vi "Plot class probabilities calculated by the VotingClassifier.vi"() -> ()   [LabVIEW 2020]
doc: "Plot the class probabilities of the first sample in a toy dataset predicted by three different classifiers and averaged by the VotingClassifier.\n\nFirst, three examplary classifiers are initialized (LogisticRegression, GaussianNB, and RandomForestClassifier) and used to initialize a soft-voting VotingClassifier with weights [1, 1, 5], which means that the predicted probabilities of the RandomForestClassifier count 5 times as much as the weights of the other classifiers when the averaged probability is calculated.\n\nTo visualize the probability weighting, we fit each classifier on the training set and plot the predicted class probabilities for the first sample in this example dataset."
uses:
  Model/Supervised/Linear_model/LinearClassifiers/LogisticRegression/LogisticRegression.lvclass
  C:/Users/cipop/TDF Dropbox/2_Technologies de France/1 - Services et Etudes/PLAIY/2 - DEV/PLAIYLAB/code/Model/Model.lvclass
  C:/Users/cipop/TDF Dropbox/2_Technologies de France/1 - Services et Etudes/PLAIY/2 - DEV/PLAIYLAB/code/Model/Supervised/Supervised.lvclass
  Model/Supervised/Ensemble/EnsembleClassifier/RandomForestClassifier/RandomForestClassifier.lvclass
  C:/Users/cipop/TDF Dropbox/2_Technologies de France/1 - Services et Etudes/PLAIY/2 - DEV/PLAIYLAB/code/Model/Supervised/Ensemble/Ensemble.lvclass
  Model/Supervised/Naive_bayes/GaussianNB/GaussianNB.lvclass
  C:/Users/cipop/TDF Dropbox/2_Technologies de France/1 - Services et Etudes/PLAIY/2 - DEV/PLAIYLAB/code/Model/Supervised/Naive_bayes/Naive_bayes.lvclass
  Model/Supervised/Linear_model/LinearClassifiers/LogisticRegression/Controls/logistic_regression_params.ctl
  Model/Supervised/Ensemble/EnsembleClassifier/RandomForestClassifier/Controls/random_forest_classifier_params.ctl
  Model/Supervised/Naive_bayes/GaussianNB/Controls/gaussian_nb_params.ctl
  Model/Supervised/Ensemble/EnsembleBlender/VotingClassifier/Controls/voting_classifier_params.ctl
  Model/Supervised/Supervised.lvclass
  Model/Supervised/Ensemble/EnsembleBlender/VotingClassifier/VotingClassifier.lvclass
  Model/Supervised/Linear_model/LinearClassifiers/LogisticRegression/LogisticRegression.vi
  Model/Supervised/Ensemble/EnsembleClassifier/RandomForestClassifier/RandomForestClassifier.vi
  Model/Supervised/Naive_bayes/GaussianNB/GaussianNB.vi
  Model/Supervised/Ensemble/EnsembleBlender/VotingClassifier/VotingClassifier.vi
panel:
  out "Plot":cluster{"X":dbl[], "Y":dbl[]}[](graph) caption="Class probabilities for sample 1 by different classifiers"
  out "error out":errorcluster
  in  "error in":errorcluster
  in  "Local":T1
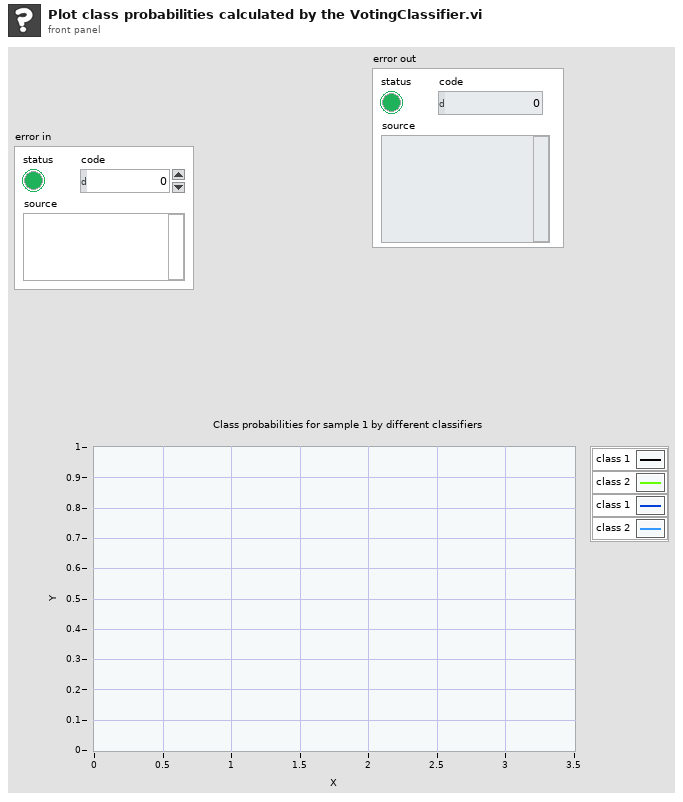
[diagram p1: front panel]
types:
  T1 = cluster{"X":dbl[][], "y":dbl[], "LogisticRegression":refnum<class "LogisticRegression.lvclass">, "RandomForestClassifier":refnum<class "RandomForestClassifier.lvclass">, "GaussianNB":refnum<class "GaussianNB.lvclass">, "clf1":dbl[][], "clf2":dbl[][], "clf3":dbl[][], "eclf":dbl[][], "class1_1":dbl[], "class2_1":dbl[], "Plot":cluster{"X":dbl[], "Y":dbl[]}[]}
  T2 = typedef "logistic_regression_params.ctl" = cluster{"penalty":string, "dual":bool, "tol":dbl, "C":dbl, "fit_intercept":bool, "intercept_scaling":dbl, "class_weight":cluster{"class_weight_type":string, "class_weight_dict":string}, "random_state":dbl, "solver":string, "max_iter":dbl, "multi_class":string, "verbose":dbl, "warm_start":bool, "n_jobs":dbl, "l1_ratio":cluster{"l1_ratio_type":string, "l1_ratio_float":dbl}}
  T3 = typedef "random_forest_classifier_params.ctl" = cluster{"n_estimators":dbl, "criterion":string, "max_depth":cluster{"max_depth_type":string, "max_depth_int":dbl}, "min_samples_split":dbl, "min_samples_leaf":dbl, "min_weight_fraction_leaf":dbl, "max_features":cluster{"max_features_type":string, "max_features_int":dbl, "max_features_float":dbl}, "max_leaf_nodes":cluster{"max_leaf_nodes_type":string, "max_leaf_nodes_int":dbl}, "min_impurity_decrease":dbl, "bootstrap":bool, "oob_score":bool, "n_jobs":dbl, "random_state":dbl, "verbose":dbl, "warm_start":bool, "class_weight":cluster{"class_weight_type":string, "class_weight_dict":string}, "ccp_alpha":dbl, "max_samples":cluster{"max_samples_type":string, "max_samples_int":dbl, "max_samples_float":dbl}}
  T4 = typedef "gaussian_nb_params.ctl" = cluster{"priors":dbl[], "var_smoothing":dbl}
  T5 = cluster{"weights_type":string, "weights_list":dbl[]}
  T6 = typedef "voting_classifier_params.ctl" = cluster{"estimators":string[], "voting":string, "weights":cluster{"weights_type":string, "weights_list":dbl[]}, "n_jobs":dbl, "flatten_transform":bool, "verbose":bool}
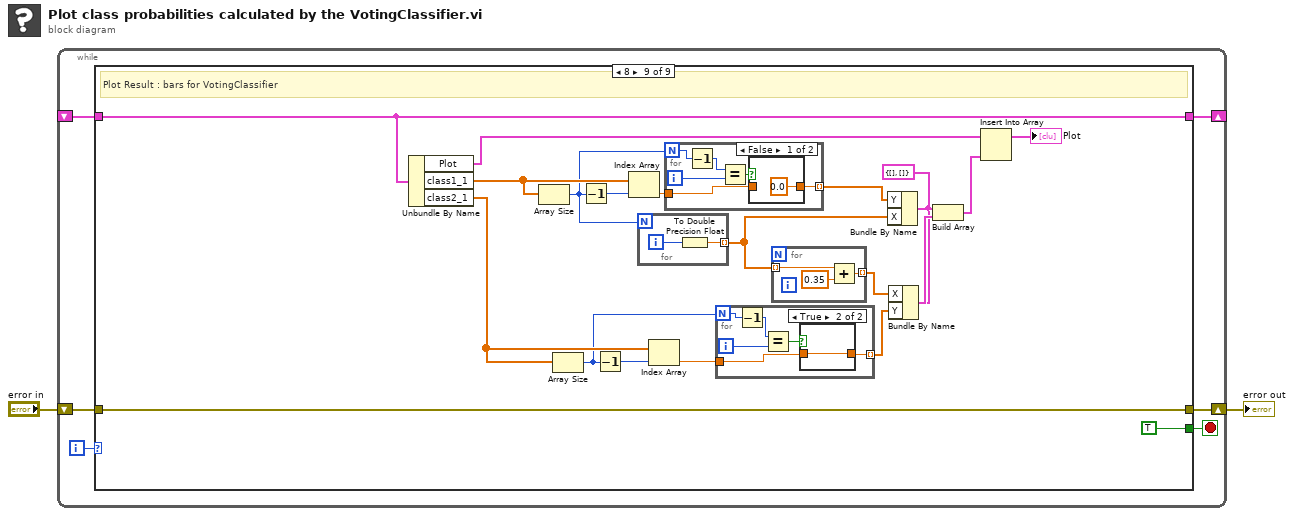
[diagram p0: block diagram]
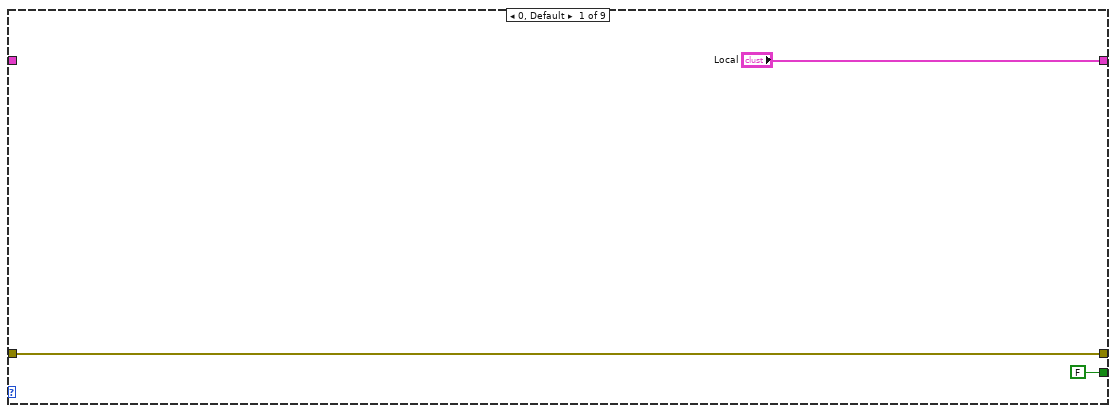
[diagram p2: hidden frame]
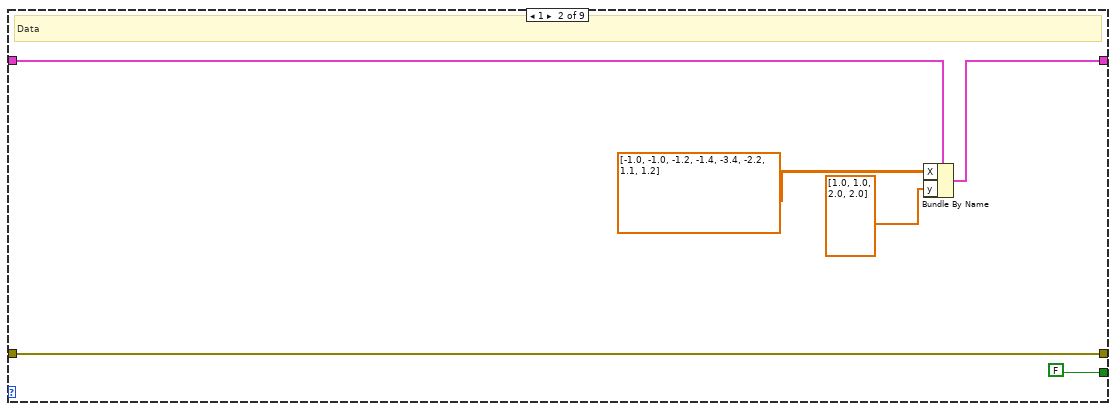
[diagram p3: hidden frame]
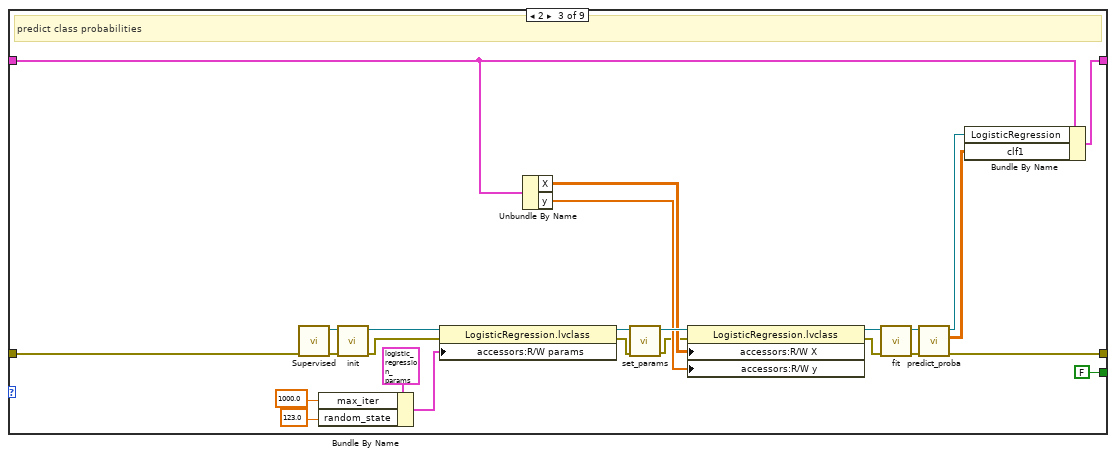
[diagram p4: hidden frame]
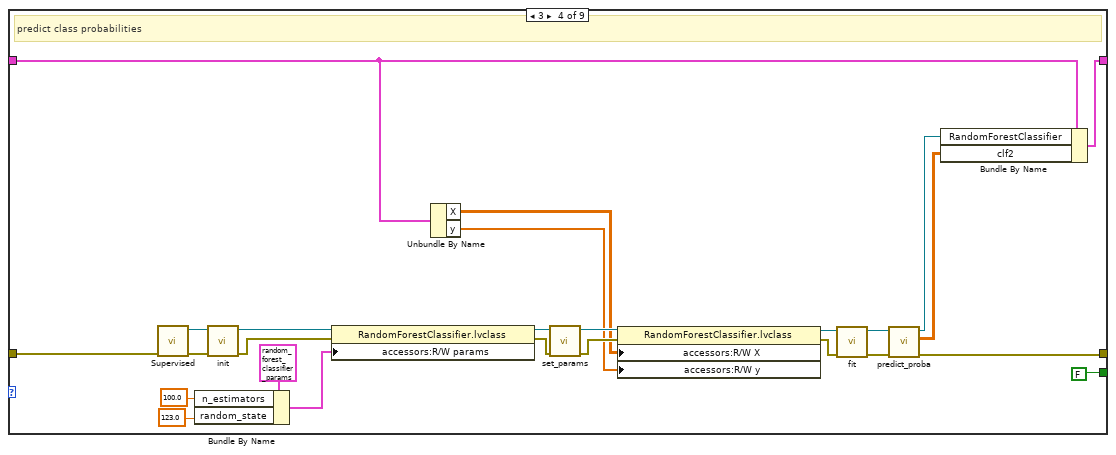
[diagram p5: hidden frame]
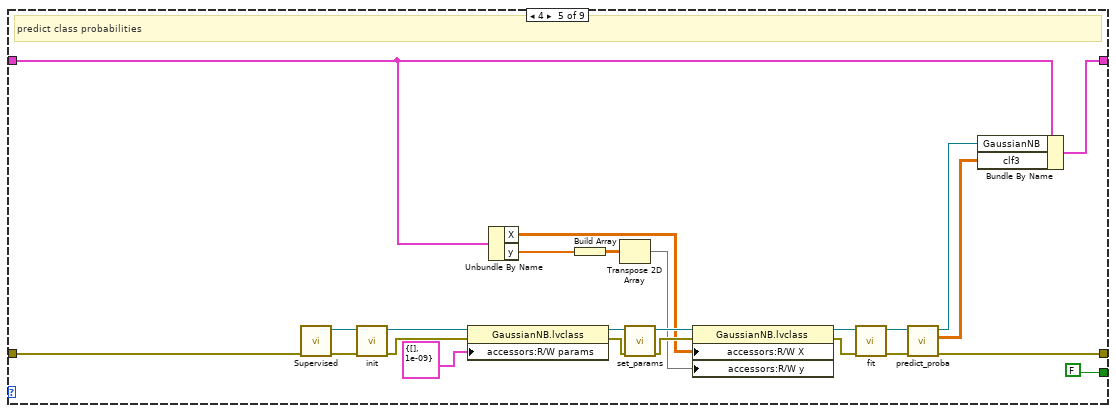
[diagram p6: hidden frame]
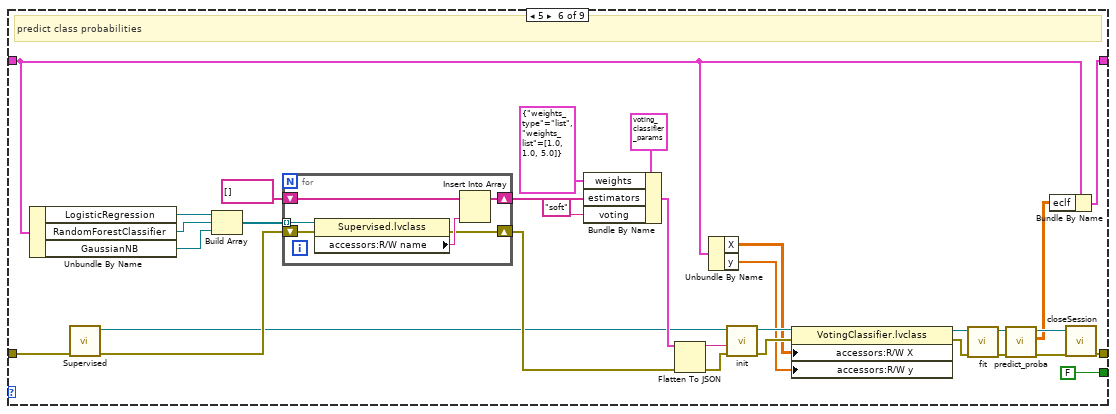
[diagram p7: hidden frame]
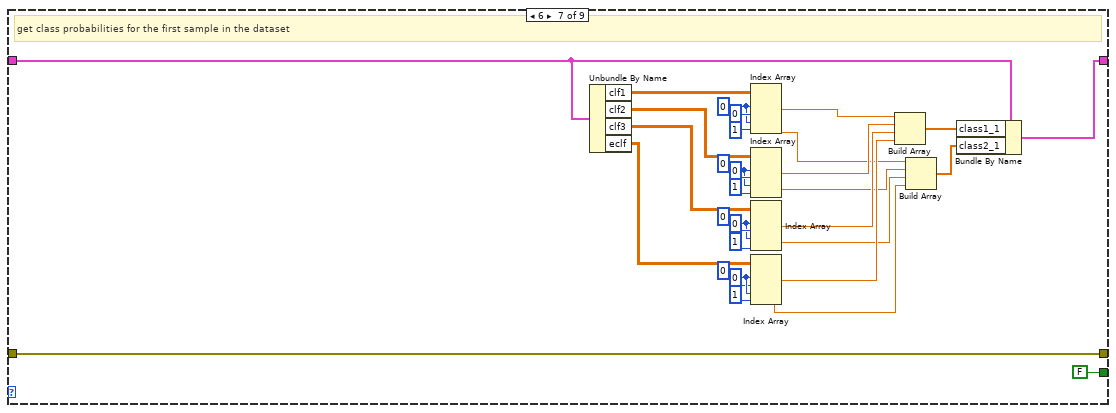
[diagram p8: hidden frame]
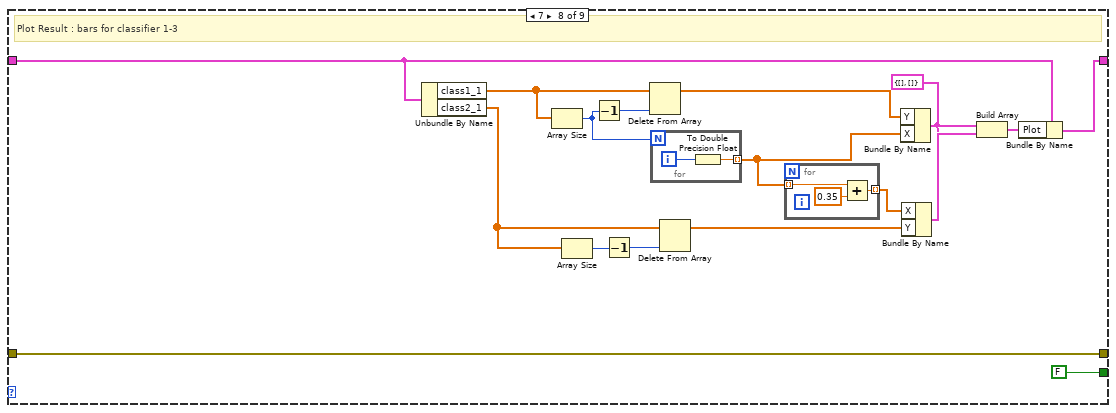
[diagram p9: hidden frame]
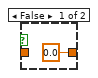
[diagram p10: hidden frame]
diagram:
  n1 = while {
    shift-right: [w6] -> w1
    shift-left: "error in" -> [w7]
    shift-right: [w5] -> _
    shift-left: _ -> [w4]
    i -> [w8]
    stop <- w3 stop-if-true
    n2 = case shown="8" w8 {
      tunnel: w7 -> [w10 w14 w36 w60 w83 w122 w133 w175 w191]
      tunnel: [w10 w14 w22 w44 w69 w117 w133 w175 w191] -> w6
      tunnel: ["Local" w15 w34 w59 w86 w94 w130 w160 w201] -> w5
      tunnel: w4 -> [_ w16 w21 w48 w79 w95 w134 w161 w201]
      tunnel: [FALSE FALSE FALSE FALSE FALSE FALSE FALSE FALSE TRUE] -> w3
      frame 0, Default {
      }
      frame 1 {
        # "Data"
        n3 = Bundle By Name(cluster=w16, "X"=dbl[][] [[-1.0, -1.0], [-1.2, -1.4], [-3.4, -2.2], [1.1, 1.2]], "y"=dbl[] [1.0, 1.0, 2.0, 2.0]) -> (w15:T1)
      }
      frame 2 {
        # "predict class probabilities"
        n4 = call-poly "Supervised.vi"("error in"=w36) -> ("error out"=w37:errorcluster, "out"=w38:refnum<class "LogisticRegression.lvclass">)  [unwired: 9 in]
        n5 = Bundle By Name(cluster=T2 {"penalty"="l2", "dual"=FALSE, "tol"=0.0001, "C"=1.0, "fit_intercept"=TRUE, "intercept_scaling"=1.0, "class_weight"={"class_weight_type"="None", "class_weight_dict"=""}, "random_state"=0.0, "solver"="lbfgs", "max_iter"=100.0, "multi_class"="auto", "verbose"=0.0, "warm_start"=FALSE, "n_jobs"=1.0, "l1_ratio"={"l1_ratio_type"="None", "l1_ratio_float"=0.0}} ("R/W params"), "max_iter"=1000.0, "random_state"=123.0) -> (w32:T2)
        n6 = call-dynamic "init.vi"("error in (no error)"=w37, "Model en entrée"=w38) -> ("error out"=w39:errorcluster, "Model en sortie"=w41:refnum<class "LogisticRegression.lvclass">)  [unwired: 8 in]
        n7 = property class="LogisticRegression.lvclass"(reference=w41, error in=w39, "accessors:R/W params"=w32) -> (reference out=w40:refnum<class "LogisticRegression.lvclass">, error out=w35:errorcluster)
        n8 = Unbundle By Name(w21) -> ("X"=w20:dbl[][], "y"=w19:dbl[])
        n9 = call-dynamic "set_params.vi"("error in (no error)"=w35, "LogisticRegression.lvclass 2"=w40) -> ("error out"=w18:errorcluster, "LogisticRegression.lvclass"=w26:refnum<class "LogisticRegression.lvclass">)  [unwired: 8 in]
        n10 = property class="LogisticRegression.lvclass"(reference=w26, error in=w18, "accessors:R/W X"=w20, "accessors:R/W y"=w19) -> (reference out=w29:refnum<class "LogisticRegression.lvclass">, error out=w25:errorcluster)
        n11 = call-dynamic "fit.vi"("error in (no error)"=w25, "LogisticRegression.lvclass 2"=w29) -> ("error out"=w27:errorcluster, "LogisticRegression.lvclass"=w28:refnum<class "LogisticRegression.lvclass">)  [unwired: 8 in]
        n12 = call-dynamic "predict_proba.vi"("error in (no error)"=w27, "LogisticRegression.lvclass 2"=w28) -> ("error out"=w22:errorcluster, "T"=w23:dbl[][], "LogisticRegression.lvclass"=w24:refnum<class "LogisticRegression.lvclass">)  [unwired: 7 in]
        n13 = Bundle By Name(cluster=w21, "LogisticRegression"=w24, "clf1"=w23) -> (w34:T1)
      }
      frame 3 {
        # "predict class probabilities"
        n14 = call-poly "Supervised.vi"("error in"=w60) -> ("error out"=w61:errorcluster, "out"=w62:refnum<class "RandomForestClassifier.lvclass">)  [unwired: 9 in]
        n15 = Bundle By Name(cluster=T3 {"n_estimators"=100.0, "criterion"="gini", "max_depth"={"max_depth_type"="None", "max_depth_int"=0.0}, "min_samples_split"=2.0, "min_samples_leaf"=1.0, "min_weight_fraction_leaf"=0.0, "max_features"={"max_features_type"="auto", "max_features_int"=0.0, "max_features_float"=0.0}, "max_leaf_nodes"={"max_leaf_nodes_type"="None", "max_leaf_nodes_int"=100.0}, "min_impurity_decrease"=0.0, "bootstrap"=TRUE, "oob_score"=FALSE, "n_jobs"=1.0, "random_state"=0.0, "verbose"=0.0, "warm_start"=FALSE, "class_weight"={"class_weight_type"="None", "class_weight_dict"="{0:1.1, 2:1.5, 2:0.6}"}, "ccp_alpha"=0.0, "max_samples"={"max_samples_type"="None", "max_samples_int"=0.0, "max_samples_float"=0.0}} ("R/W params"), "n_estimators"=100.0, "random_state"=123.0) -> (w55:T3)
        n16 = call-dynamic "init.vi"("error in (no error)"=w61, "Model en entrée"=w62) -> ("error out"=w64:errorcluster, "Model en sortie"=w66:refnum<class "RandomForestClassifier.lvclass">)  [unwired: 8 in]
        n17 = property class="RandomForestClassifier.lvclass"(reference=w66, error in=w64, "accessors:R/W params"=w55) -> (reference out=w65:refnum<class "RandomForestClassifier.lvclass">, error out=w63:errorcluster)
        n18 = Unbundle By Name(w48) -> ("X"=w47:dbl[][], "y"=w46:dbl[])
        n19 = call-dynamic "set_params.vi"("error in (no error)"=w63, "RandomForestClassifier.lvclass 2"=w65) -> ("error out"=w50:errorcluster, "RandomForestClassifier.lvclass"=w51:refnum<class "RandomForestClassifier.lvclass">)  [unwired: 8 in]
        n20 = property class="RandomForestClassifier.lvclass"(reference=w51, error in=w50, "accessors:R/W X"=w47, "accessors:R/W y"=w46) -> (reference out=w54:refnum<class "RandomForestClassifier.lvclass">, error out=w49:errorcluster)
        n21 = call-dynamic "fit.vi"("error in (no error)"=w49, "Ensemble.lvclass 2"=w54) -> ("error out"=w52:errorcluster, "Ensemble.lvclass"=w53:refnum<class "RandomForestClassifier.lvclass">)  [unwired: 8 in]
        n22 = call-dynamic "predict_proba.vi"("error in (no error)"=w52, "EnsembleClassifier.lvclass 2"=w53) -> ("error out"=w44:errorcluster, "T"=w43:dbl[][], "EnsembleClassifier.lvclass"=w45:refnum<class "RandomForestClassifier.lvclass">)  [unwired: 7 in]
        n23 = Bundle By Name(cluster=w48, "RandomForestClassifier"=w45, "clf2"=w43) -> (w59:T1)
      }
      frame 4 {
        # "predict class probabilities"
        n24 = call-poly "Supervised.vi"("error in"=w83) -> ("error out"=w84:errorcluster, "out"=w85:refnum<class "GaussianNB.lvclass">)  [unwired: 9 in]
        n25 = call-dynamic "init.vi"("error in (no error)"=w84, "Model en entrée"=w85) -> ("error out"=w88:errorcluster, "Model en sortie"=w90:refnum<class "GaussianNB.lvclass">)  [unwired: 8 in]
        n26 = property class="GaussianNB.lvclass"(reference=w90, error in=w88, "accessors:R/W params"=T4 {"priors"=[], "var_smoothing"=1e-09} ("R/W params")) -> (reference out=w89:refnum<class "GaussianNB.lvclass">, error out=w87:errorcluster)
        n27 = Unbundle By Name(w79) -> ("X"=w78:dbl[][], "y"=w77:dbl[])
        n28 = Build Array(w77) -> (w76:dbl[][])
        n29 = Transpose 2D Array(2D array=w76) -> (transposed array=w75:dbl[][])
        n30 = call-dynamic "set_params.vi"("error in (no error)"=w87, "GaussianNB.lvclass 2"=w89) -> ("error out"=w80:errorcluster, "GaussianNB.lvclass"=w81:refnum<class "GaussianNB.lvclass">)  [unwired: 8 in]
        n31 = property class="GaussianNB.lvclass"(reference=w81, error in=w80, "accessors:R/W X"=w78, "accessors:R/W y"=w75) -> (reference out=w74:refnum<class "GaussianNB.lvclass">, error out=w73:errorcluster)
        n32 = call-dynamic "fit.vi"("error in (no error)"=w73, "Naive_bayes.lvclass 2"=w74) -> ("error out"=w71:errorcluster, "Naive_bayes.lvclass"=w72:refnum<class "GaussianNB.lvclass">)  [unwired: 8 in]
        n33 = call-dynamic "predict_proba.vi"("error in (no error)"=w71, "Naive_bayes.lvclass 2"=w72) -> ("error out"=w69:errorcluster, "T"=w68:dbl[][], "Naive_bayes.lvclass"=w70:refnum<class "GaussianNB.lvclass">)  [unwired: 7 in]
        n34 = Bundle By Name(cluster=w79, "GaussianNB"=w70, "clf3"=w68) -> (w86:T1)
      }
      frame 5 {
        # "predict class probabilities"
        n35 = Unbundle By Name(w95) -> ("LogisticRegression"=w110:refnum<class "LogisticRegression.lvclass">, "RandomForestClassifier"=w109:refnum<class "RandomForestClassifier.lvclass">, "GaussianNB"=w119:refnum<class "GaussianNB.lvclass">)
        n36 = call-poly "Supervised.vi"("error in"=w122) -> ("error out"=w115:errorcluster, "out"=w108:refnum<class "VotingClassifier.lvclass">)  [unwired: 9 in]
        n37 = Build Array(w110, w109, w119) -> (w121:refnum<class "Supervised.lvclass">[])
        n38 = for {
          tunnel: w121 -> [w125] mode=indexing
          shift-right: [w126] -> w116
          shift-left: string[] [] -> [w128]
          shift-right: [w123] -> w113
          shift-left: w115 -> [w124]
          n39 = property class="Supervised.lvclass"(reference=w125, error in=w124) -> (error out=w123:errorcluster, "accessors:R/W name"=w127:string)  [unwired: 1 out]
          n40 = Insert Into Array(array=w128, new element=w127) -> (w126:string[])  [unwired: 1 in]
        }
        n41 = Bundle By Name(cluster=T6 {"estimators"=[], "voting"="hard", "weights"={"weights_type"="None", "weights_list"=[]}, "n_jobs"=1.0, "flatten_transform"=TRUE, "verbose"=FALSE} ("R/W params"), "weights"=T5 {"weights_type"="list", "weights_list"=[1.0, 1.0, 5.0]}, "estimators"=w116, "voting"="soft") -> (w114:T6)
        n42 = Flatten To JSON(anything=w114, error in (no error)=w113) -> (JSON string=w111:string, 11:w112:errorcluster)  [unwired: 1 in]
        n43 = Unbundle By Name(w95) -> ("X"=w98:dbl[][], "y"=w97:dbl[])
        n44 = call-dynamic "init.vi"("error in (no error)"=w112, "json of params"=w111, "EnsembleBlender in"=w108) -> ("error out"=w102:errorcluster, "EnsembleBlender out"=w103:refnum<class "VotingClassifier.lvclass">)  [unwired: 7 in]
        n45 = property class="VotingClassifier.lvclass"(reference=w103, error in=w102, "accessors:R/W X"=w98, "accessors:R/W y"=w97) -> (reference out=w101:refnum<class "VotingClassifier.lvclass">, error out=w105:errorcluster)
        n46 = call-dynamic "fit.vi"("error in (no error)"=w105, "Ensemble.lvclass 2"=w101) -> ("error out"=w104:errorcluster, "Ensemble.lvclass"=w96:refnum<class "VotingClassifier.lvclass">)  [unwired: 8 in]
        n47 = call-dynamic "predict_proba.vi"("error in (no error)"=w104, "VotingClassifier in"=w96) -> ("error out"=w99:errorcluster, "T"=w93:dbl[][], "VotingClassifier out"=w100:refnum<class "VotingClassifier.lvclass">)  [unwired: 7 in]
        n48 = Bundle By Name(cluster=w95, "eclf"=w93) -> (w94:T1)
        n49 = call-dynamic "closeSession.vi"("error in"=w99, "Python en entrée"=w100) -> ("error out"=w117:errorcluster)  [unwired: 8 in, 1 out]
      }
      frame 6 {
        w137 = 0 ("disabled index (row)")
        w140 = 0 ("disabled index (row)")
        w143 = 0 ("disabled index (row)")
        w146 = 0 ("disabled index (row)")
        # "get class probabilities for the first sample in the dataset"
        n50 = Unbundle By Name(w134) -> ("clf1"=w158:dbl[][], "clf2"=w155:dbl[][], "clf3"=w153:dbl[][], "eclf"=w151:dbl[][])
        n51 = Index Array(array=w158, index (row) #1=w146, index (col) #1=0 ("disabled index (col)"), index (row) #2=w146, index (col) #2=1 ("disabled index (col)")) -> (element #1=w150:dbl, element #2=w144:dbl)
        n52 = Index Array(array=w155, index (row) #1=w143, index (col) #1=0 ("disabled index (col)"), index (row) #2=w143, index (col) #2=1 ("disabled index (col)")) -> (element #1=w149:dbl, element #2=w141:dbl)
        n53 = Index Array(array=w153, index (row) #1=w140, index (col) #1=0 ("disabled index (col)"), index (row) #2=w140, index (col) #2=1 ("disabled index (col)")) -> (element #1=w148:dbl, element #2=w138:dbl)
        n54 = Index Array(array=w151, index (row) #1=w137, index (col) #1=0 ("disabled index (col)"), index (row) #2=w137, index (col) #2=1 ("disabled index (col)")) -> (element #1=w147:dbl, element #2=w135:dbl)
        n55 = Build Array(w150, w149, w148, w147) -> (w132:dbl[])
        n56 = Build Array(w144, w141, w138, w135) -> (w131:dbl[])
        n57 = Bundle By Name(cluster=w134, "class1_1"=w132, "class2_1"=w131) -> (w130:T1)
      }
      frame 7 {
        w167 = cluster{"X":dbl[], "Y":dbl[]} {"X"=[], "Y"=[]} ("Cluster")
        # "Plot Result : bars for classifier 1-3"
        n58 = Unbundle By Name(w161) -> ("class1_1"=w168:dbl[], "class2_1"=w166:dbl[])
        n59 = Array Size(array=w168) -> (size(s)=w163:i32)
        n60 = Array Size(array=w166) -> (size(s)=w172:i32)
        n61 = Decrement(x=w163) -> (x-1=w162:i32)
        n62 = Decrement(x=w172) -> (x-1=w165:i32)
        n63 = Delete From Array(array=w168, index=w162) -> (array with subset deleted=w174:dbl[])  [unwired: 1 in, 1 out]
        n64 = for {
          N: w163 -> [_]
          tunnel: [w180] -> w169 mode=indexing
          i -> [w181]
          n65 = To Double Precision Float(number=w181) -> (double precision float=w180:dbl)
        }
        n66 = Delete From Array(array=w166, index=w165) -> (array with subset deleted=w171:dbl[])  [unwired: 1 in, 1 out]
        n67 = for {
          tunnel: w169 -> [w179] mode=indexing
          tunnel: [w177] -> w164 mode=indexing
          n68 = Add(x=w179, y=0.35) -> (x+y=w177:dbl)
        }
        n69 = Bundle By Name(cluster=w167, "Y"=w174, "X"=w169) -> (w173:cluster{"X":dbl[], "Y":dbl[]})
        n70 = Bundle By Name(cluster=w167, "X"=w164, "Y"=w171) -> (w170:cluster{"X":dbl[], "Y":dbl[]})
        n71 = Build Array(w173, w170) -> (w159:cluster{"X":dbl[], "Y":dbl[]}[])
        n72 = Bundle By Name(cluster=w161, "Plot"=w159) -> (w160:T1)
      }
      frame 8 {
        w196 = cluster{"X":dbl[], "Y":dbl[]} {"X"=[], "Y"=[]} ("Cluster")
        # "Plot Result : bars for VotingClassifier"
        n73 = Unbundle By Name(w201) -> ("Plot"=w190:cluster{"X":dbl[], "Y":dbl[]}[], "class1_1"=w197:dbl[], "class2_1"=w195:dbl[])
        n74 = Array Size(array=w197) -> (size(s)=w187:i32)
        n75 = Array Size(array=w195) -> (size(s)=w182:i32)
        n76 = Decrement(x=w187) -> (x-1=w192:i32)
        n77 = Decrement(x=w182) -> (x-1=w194:i32)
        n78 = Index Array(array=w197, index=w192) -> (element=w186:dbl)
        n79 = for {
          N: w187 -> [_]
          tunnel: [w222] -> w198 mode=indexing
          i -> [w223]
          n80 = To Double Precision Float(number=w223) -> (double precision float=w222:dbl)
        }
        n81 = Index Array(array=w195, index=w194) -> (element=w183:dbl)
        n82 = for {
          N: w187 -> [w213]
          tunnel: w186 -> [w215]
          tunnel: [w214] -> w185 mode=indexing
          i -> [w211]
          n83 = Decrement(x=w213) -> (x-1=w212:i32)
          n84 = Equal?(x=w212, y=w211) -> (x = y?=w216:bool)
          n85 = case shown="False" w216 {
            tunnel: w215 -> [_ w218]
            tunnel: [0.0 ("Numeric") w218] -> w214
            frame False {
            }
            frame True {
            }
          }
        }
        n86 = for {
          N: w182 -> [w205]
          tunnel: w183 -> [w207]
          tunnel: [w206] -> w184 mode=indexing
          i -> [w203]
          n87 = Decrement(x=w205) -> (x-1=w204:i32)
          n88 = Equal?(x=w204, y=w203) -> (x = y?=w208:bool)
          n89 = case shown="True" w208 {
            tunnel: w207 -> [_ w210]
            tunnel: [0.0 ("Numeric") w210] -> w206
            frame False {
            }
            frame True {
            }
          }
        }
        n90 = for {
          tunnel: w198 -> [w221] mode=indexing
          tunnel: [w219] -> w193 mode=indexing
          n91 = Add(x=w221, y=0.35) -> (x+y=w219:dbl)
        }
        n92 = Bundle By Name(cluster=w196, "Y"=w185, "X"=w198) -> (w200:cluster{"X":dbl[], "Y":dbl[]})
        n93 = Bundle By Name(cluster=w196, "X"=w193, "Y"=w184) -> (w199:cluster{"X":dbl[], "Y":dbl[]})
        n94 = Build Array(w200, w199) -> (w189:cluster{"X":dbl[], "Y":dbl[]}[])
        n95 = Insert Into Array(array=w190, new element=w189) -> (→"Plot":cluster{"X":dbl[], "Y":dbl[]}[])  [unwired: 1 in]
      }
    }
  }
  "error out" <- w1
